vi "模拟量采集.vi"(10 "数据数组":dbl[][](array[numeric]) caption="二维数组") -> (0 "齿条推拉力":dbl format="%#_2f", 1 "间隙位移":dbl format="%#_2f", 2 "调整螺塞扭矩":dbl format="%#_3f", 3 "齿条扭矩":dbl format="%#_2f")   [LabVIEW 2013]
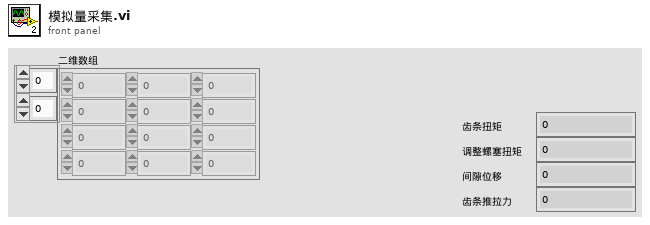
[diagram p1: front panel]
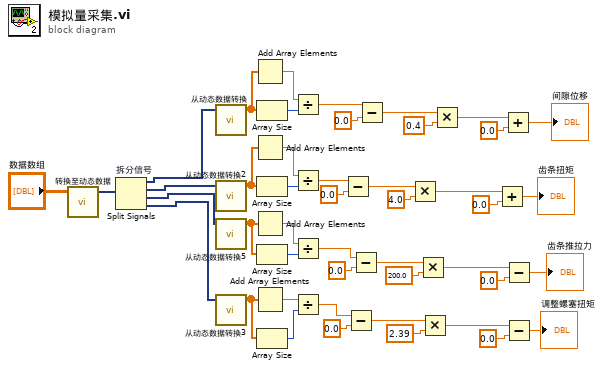
[diagram p0: block diagram]
diagram:
  n1 = call "转换至动态数据"("2D Array"="数据数组") -> ("Dynamic Data Type"=w9:dynamicdata)  [unwired: 3 in]
  n2 = Split Signals "拆分信号"(w9) -> (w8:dynamicdata, w7:dynamicdata, w6:dynamicdata, w5:dynamicdata)  [unwired: 4 in]
  n3 = call "从动态数据转换"("Dynamic Data Type"=w8) -> ("Array"=w46:dbl[])  [unwired: 3 in]
  n4 = call "从动态数据转换2"("Dynamic Data Type"=w7) -> ("Array"=w43:dbl[])  [unwired: 3 in]
  n5 = call "从动态数据转换5"("Dynamic Data Type"=w6) -> ("Array"=w20:dbl[])  [unwired: 3 in]
  n6 = call "从动态数据转换3"("Dynamic Data Type"=w5) -> ("Array"=w40:dbl[])  [unwired: 3 in]
  n7 = Add Array Elements(numeric array=w46) -> (sum=w45:dbl)
  n8 = Add Array Elements(numeric array=w43) -> (sum=w42:dbl)
  n9 = Add Array Elements(numeric array=w20) -> (sum=w19:dbl)
  n10 = Add Array Elements(numeric array=w40) -> (sum=w39:dbl)
  n11 = Array Size(array=w46) -> (size(s)=w44:i32)
  n12 = Array Size(array=w43) -> (size(s)=w41:i32)
  n13 = Array Size(array=w20) -> (size(s)=w18:i32)
  n14 = Array Size(array=w40) -> (size(s)=w38:i32)
  n15 = Divide(x=w45, y=w44) -> (x/y=w1:dbl)
  n16 = Divide(x=w42, y=w41) -> (x/y=w2:dbl)
  n17 = Divide(x=w19, y=w18) -> (x/y=w4:dbl)
  n18 = Divide(x=w39, y=w38) -> (x/y=w3:dbl)
  n19 = Subtract(x=w2, y=0.0) -> (x-y=w25:dbl)
  n20 = Subtract(x=w3, y=0.0) -> (x-y=w23:dbl)
  n21 = Subtract(x=w4, y=0.0) -> (x-y=w21:dbl)
  n22 = Subtract(x=w1, y=0.0) -> (x-y=w13:dbl)
  n23 = Multiply(x=w25, y=4.0) -> (x*y=w37:dbl)
  n24 = Multiply(x=w21, y=200.0) -> (x*y=w31:dbl)
  n25 = Multiply(x=w23, y=2.39) -> (x*y=w34:dbl)
  n26 = Multiply(x=w13, y=0.4) -> (x*y=w17:dbl)
  n27 = Add(x=w37, y=0.0) -> (x+y=→"齿条扭矩":dbl)
  n28 = Add(x=w17, y=0.0) -> (x+y=→"间隙位移":dbl)
  n29 = Subtract(x=w31, y=0.0) -> (x-y=→"齿条推拉力":dbl)
  n30 = Subtract(x=w34, y=0.0) -> (x-y=→"调整螺塞扭矩":dbl)
